vi "Get Name.vi"(8 "error in":errorcluster, 11 "Device Profile in":refnum<class "Device Profile.lvclass">) -> (0 "error out":errorcluster, 2 "Name":string, 3 "Device Profile out":refnum<class "Device Profile.lvclass">)   [LabVIEW 2020, in "CANopen.lvlib" / "Device Profile.lvclass"]
uses:
  Device Profile.lvclass
  Device Profile.lvclass/Device Profile.ctl
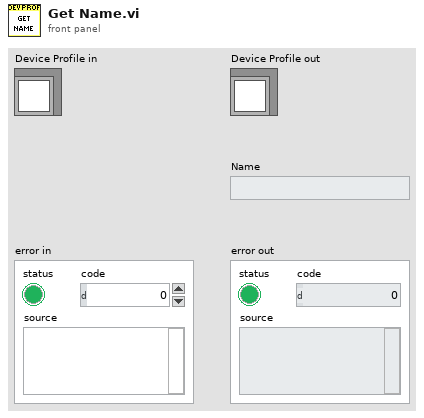
[diagram p1: front panel]
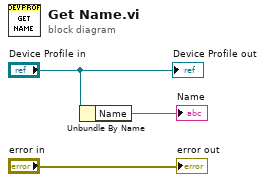
[diagram p0: block diagram]
diagram:
  n1 = Unbundle By Name("Device Profile in") -> ("Name"=→"Name":string)
  "error out" <- "error in"
  "Device Profile out" <- "Device Profile in"
